vi "directoryTest.vi"() -> ()   [LabVIEW 2016]
panel:
  out "return code 2":i32
  out "standard error 2":string
  out "standard output 2":string
  out "error out":errorcluster
  out "return code":i32
  out "standard error":string
  out "standard output":string
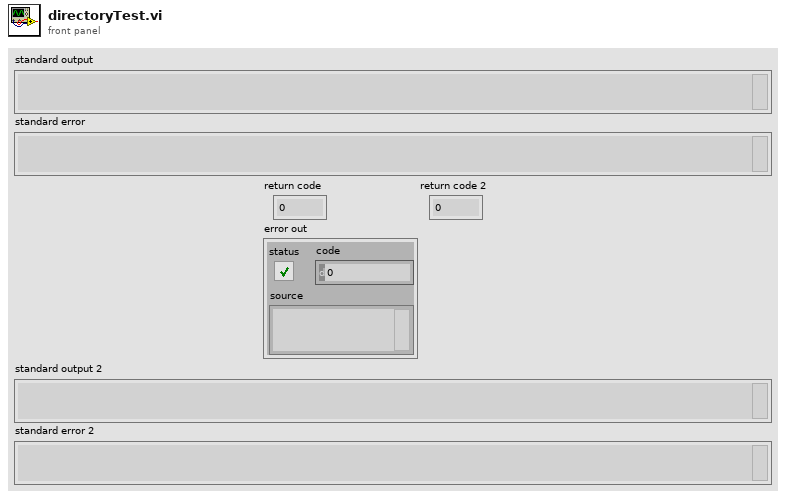
[diagram p1: front panel]
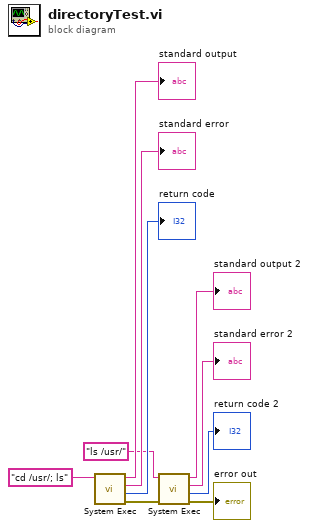
[diagram p0: block diagram]
diagram:
  n1 = call <vilib>:"System Exec.vi"("command line"="cd /usr/; ls") -> ("error out"=w6:errorcluster, "return code"=→"return code":i32, "standard error"=→"standard error":string, "standard output"=→"standard output":string)  [unwired: 7 in]
  n2 = call <vilib>:"System Exec.vi"("error in (no error)"=w6, "command line"="ls /usr/") -> ("error out"=→"error out":errorcluster, "return code"=→"return code 2":i32, "standard error"=→"standard error 2":string, "standard output"=→"standard output 2":string)  [unwired: 6 in]
